vi "Request Immediate Session Disconnection.vi"(8 "error in (no error)":errorcluster, 9 "Protocol Violation Error Code":i32, 10 "Disconnection Reason":T1, 11 "Session in":refnum<class "Session.lvclass">) -> (0 "error out":errorcluster, 3 "Session out":refnum<class "Session.lvclass">)   [LabVIEW 2013, in "MQTT Base.lvlib" / "Session.lvclass"]
uses:
  Session.lvclass
  Session Disconnection Reason -- enum.ctl
  Base Class/Response -- cluster.ctl
  <vilib>/LabVIEW Open Source Project/MQTT Control Packets/Control Packets/ControlPacket/ControlPacket.lvclass
  Session.lvclass/Session.ctl
  Base Class/MQTT_Base.lvclass
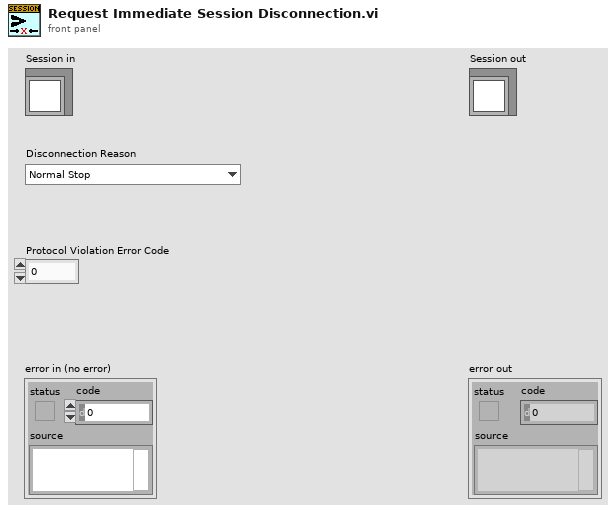
[diagram p1: front panel]
types:
  T1 = typedef "MQTT Base.lvlib/Session.lvclass/Session Disconnection Reason -- enum.ctl" = enum16{"Normal Stop", "Protocol Violation", "Disconnected by Peer"}
  T2 = typedef "MQTT Base.lvlib/MQTT_Base.lvclass/Response -- cluster.ctl" = cluster{"Packet":refnum<class "ControlPacket.lvclass">, "Protocol Error":errorcluster, "disconnect session":bool, "[ACK]":refnum<notifier>[]}
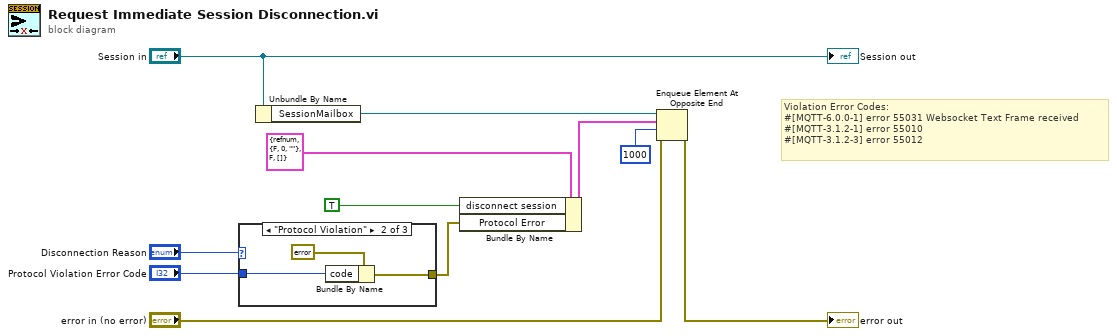
[diagram p0: block diagram]
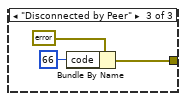
[diagram p3: hidden frame]
diagram:
  # "Violation Error Codes: \n#[MQTT-6.0.0-1] error 55031 Websocket Text Frame received\n#[MQTT-3.1.2-1] error 55010\n#[MQTT-3.1.2-3] error 55012"
  n1 = case shown="\"Protocol Violation\"" "Disconnection Reason" {
    tunnel: "Protocol Violation Error Code" -> [_ w13 _]
    tunnel: [_ w12 w16] -> w1
    frame "Normal Stop", Default {
    }
    frame "Protocol Violation" {
      n2 = Bundle By Name(cluster=errorcluster {"status"=TRUE, "code"=0, "source"=""} ("Protocol Error"), "code"=w13) -> (w12:errorcluster)
    }
    frame "Disconnected by Peer" {
      n3 = Bundle By Name(cluster=errorcluster {"status"=TRUE, "code"=0, "source"=""} ("Protocol Error"), "code"=66) -> (w16:errorcluster)
    }
  }
  n4 = Unbundle By Name("Session in") -> ("SessionMailbox"=w6:refnum<queue>)
  n5 = Bundle By Name(cluster=T2 {"Packet"=refnum, "Protocol Error"={"status"=FALSE, "code"=0, "source"=""}, "disconnect session"=FALSE, "[ACK]"=[]} ("element"), "disconnect session"=TRUE, "Protocol Error"=w1) -> (w3:T2)
  n6 = Enqueue Element At Opposite End(queue=w6, element=w3, timeout in ms (-1)=1000, error in (no error)="error in (no error)") -> (error out=→"error out":errorcluster)  [unwired: 2 out]
  "Session out" <- "Session in"
